vi "LoadItemValuesFromFile_Simple.vi"(0 "Array in":string[][](array[string]), 5 "FileArray":string[](array[string]), 11 "error in (no error)":errorcluster) -> (3 "Values":dbl[][](array[numeric]), 4 "Item":string[](array[string]), 6 "Time 60/min":dbl[](array[numeric]), 15 "error out":errorcluster)   [LabVIEW 2018]
doc: "Each row of the input string array specifies the Item, Dataset, Group, and Filepath of the data to be queried.\nUse these strings to look up the relevant data within the HDF5 records. The output values and corresponding TimeString or Timestamp arrays are suitable for plotting.\n\nItem (MaxValue, PeakLoc, etc.)\nDataset (Beac, Cal, etc.)\nGroup (84GHz_Cross, 72GHz_Cross, etc.)\nFile (filename of the HDF5 file)"
uses:
  <vilib>/addons/h5labview2/file/H5Fmode.ctl
  HDF5/lib_path_mod_20200519.vi
  <vilib>/addons/h5labview2/base/H5Equery.vi
  <vilib>/addons/h5labview2/attrib/H5Aread.llb/H5Aread.xnode
  <vilib>/addons/h5labview2/dataset/H5Dread.llb/H5Dread.xnode
  <vilib>/addons/h5labview2/file/H5F.lvlib
  <vilib>/addons/h5labview2/group/H5G.lvlib
  <vilib>/addons/h5labview2/dataset/H5D.lvlib
panel:
  out "UseFastRate":bool
  out "Time 1/min":dbl[](array[numeric])
  # "Item"
  # "Dataset"
  # "Group"
  # "Filepath"
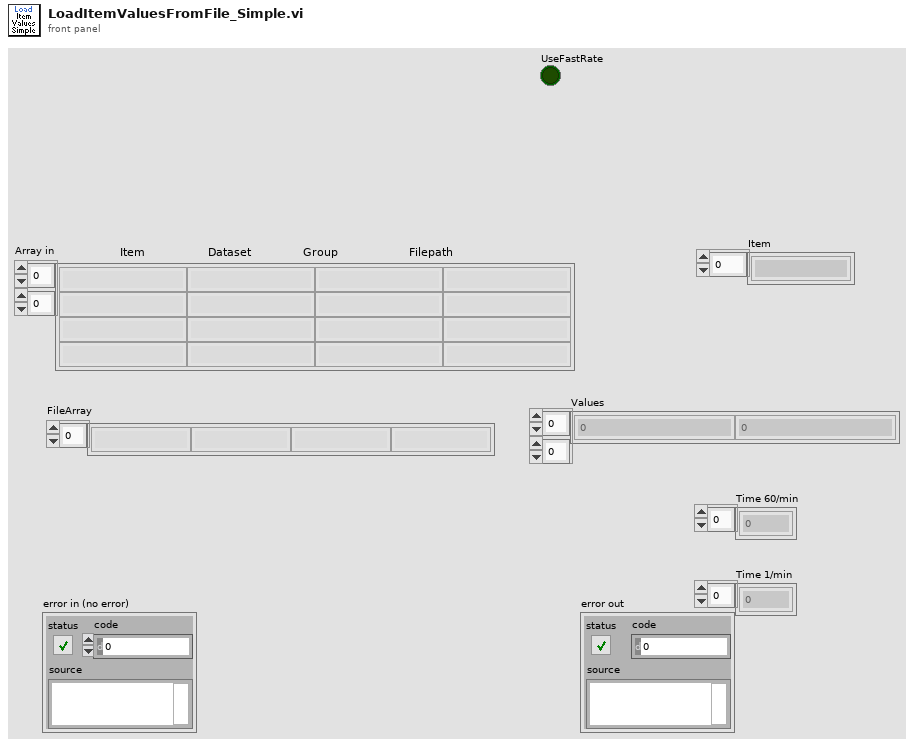
[diagram p1: front panel]
types:
  T1 = typedef "H5F.lvlib/H5Fmode.ctl" = enum16{"read-only", "read-write", "overwrite", "create new", "open or create"}
  T2 = typedef "hid_t.ctl" = i32
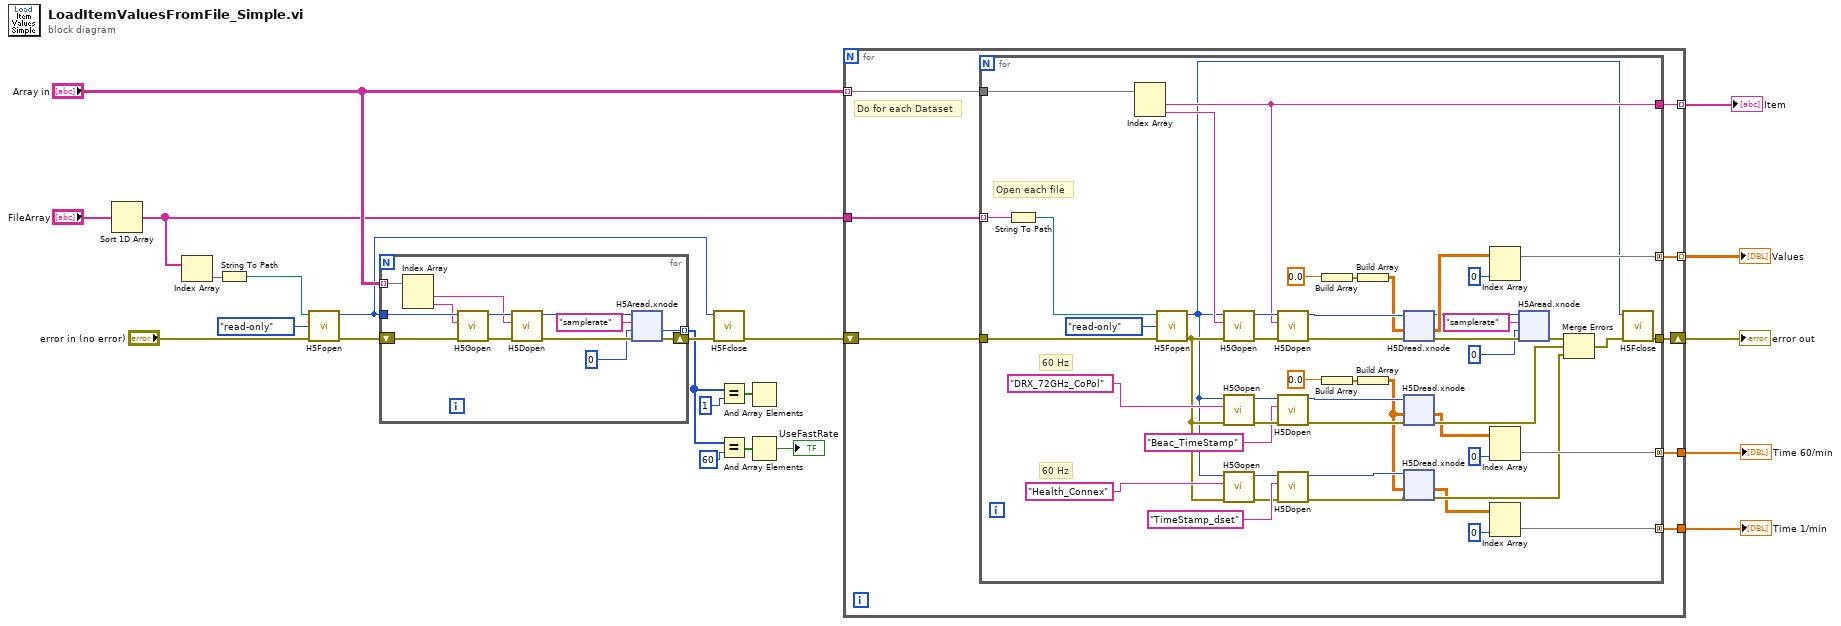
[diagram p0: block diagram]
diagram:
  n1 = Sort 1D Array(array="FileArray") -> (sorted array=w1:string[])
  n2 = Index Array(array=w1) -> (element=w15:string)  [unwired: 1 in]
  n3 = String To Path(string=w15) -> (path=w14:path)
  n4 = call <vilib>:"H5Fopen.vi"("error in (no error)"="error in (no error)", "mode (read-only)"=H5Fmode."read-only" ("mode"), "path"=w14) -> ("error out"=w11:errorcluster, "ref out"=w2:T2)  [unwired: 7 in]
  n5 = for {
    tunnel: w2 -> [w34]
    shift-right: [w28] -> w10
    shift-left: w11 -> [w31]
    tunnel: [w26] -> w7 mode=indexing
    tunnel: "Array in" -> [w25] mode=indexing
    n6 = Index Array(array=w25) -> (element #1=w23:string, element #2=w24:string)  [unwired: 2 in]
    n7 = call <vilib>:"H5Gopen.vi"("error in (no error)"=w31, "name"=w24, "ref in"=w34) -> ("error out"=w30:errorcluster, "group out"=w33:T2)  [unwired: 7 in]
    n8 = call <vilib>:"H5Dopen.vi"("error in (no error)"=w30, "name"=w23, "loc in"=w33) -> ("error out"=w29:errorcluster, "dset out"=w32:T2)  [unwired: 7 in]
    n9 = xnode "H5Aread.xnode"("error in (no error)"=w29, "default"=u32 0, "attrib name"="samplerate", "ref in"=w32) -> ("error out"=w28:errorcluster, "data"=w26:u32)  [unwired: 2 in, 2 out]
  }
  n10 = call <vilib>:"H5Fclose.vi"("error in (no error)"=w10, "ref"=w2) -> ("error out"=w13:errorcluster)  [unwired: 9 in]
  n11 = Equal?(x=w7, y=u32 1 ("data")) -> (x = y?=w5:bool[])
  n12 = Equal?(x=w7, y=u32 60 ("data")) -> (x = y?=w6:bool[])
  n13 = And Array Elements(Boolean array=w5) -> ()  [unwired: 1 out]
  n14 = And Array Elements(Boolean array=w6) -> (logical AND=→"UseFastRate":bool)
  n15 = for {
    tunnel: w1 -> [w58]
    tunnel: [w56] -> w21 mode=indexing
    shift-right: [w57] -> w22
    shift-left: w13 -> [w52]
    tunnel: [w55] -> w20
    tunnel: "Array in" -> [w54] mode=indexing
    tunnel: [w53] -> w19 mode=indexing
    tunnel: [w51] -> w18
    # "Do for each Dataset"
    n16 = for {
      tunnel: w58 -> [w106] mode=indexing
      tunnel: [w100] -> w57
      tunnel: [w94] -> w56 mode=concatenating
      tunnel: [w83] -> w55 mode=concatenating
      tunnel: w54 -> [w82]
      tunnel: [w80] -> w53
      tunnel: w52 -> [w79]
      tunnel: [w76] -> w51 mode=concatenating
      # "60 Hz"
      # "60 Hz"
      # "Open each file"
      n17 = String To Path(string=w106) -> (path=w105:path)
      n18 = Index Array(array=w82) -> (element #1=w80:string, element #2=w81:string)  [unwired: 2 in]
      n19 = call <vilib>:"H5Fopen.vi"("error in (no error)"=w79, "mode (read-only)"=H5Fmode."read-only" ("mode"), "path"=w105) -> ("error out"=w70:errorcluster, "ref out"=w68:T2)  [unwired: 7 in]
      n20 = call <vilib>:"H5Gopen.vi"("error in (no error)"=w70, "name"=w81, "ref in"=w68) -> ("error out"=w102:errorcluster, "group out"=w104:T2)  [unwired: 7 in]
      n21 = call <vilib>:"H5Gopen.vi"("error in (no error)"=w70, "name"="DRX_72GHz_CoPol", "ref in"=w68) -> ("error out"=w90:errorcluster, "group out"=w88:T2)  [unwired: 7 in]
      n22 = call <vilib>:"H5Gopen.vi"("error in (no error)"=w70, "name"="Health_Connex", "ref in"=w68) -> ("error out"=w71:errorcluster, "group out"=w72:T2)  [unwired: 7 in]
      n23 = call <vilib>:"H5Dopen.vi"("error in (no error)"=w102, "name"=w80, "loc in"=w104) -> ("error out"=w101:errorcluster, "dset out"=w103:T2)  [unwired: 7 in]
      n24 = call <vilib>:"H5Dopen.vi"("error in (no error)"=w90, "name"="Beac_TimeStamp", "loc in"=w88) -> ("error out"=w91:errorcluster, "dset out"=w89:T2)  [unwired: 7 in]
      n25 = call <vilib>:"H5Dopen.vi"("error in (no error)"=w71, "name"="TimeStamp_dset", "loc in"=w72) -> ("error out"=w69:errorcluster, "dset out"=w67:T2)  [unwired: 7 in]
      n26 = Build Array(0.0 ("HDF5_ToneInfo in")) -> (w99:dbl[])
      n27 = Build Array(0.0 ("HDF5_ToneInfo in")) -> (w92:dbl[])
      n28 = Build Array(w99) -> (w98:dbl[][])
      n29 = Build Array(w92) -> (w66:dbl[][])
      n30 = xnode "H5Dread.xnode"("error in (no error)"=w101, "default"=w98, "ref in"=w103) -> ("error out"=w62:errorcluster, "data"=w96:dbl[][], "ref out"=w63:i32)  [unwired: 3 in, 1 out]
      n31 = xnode "H5Dread.xnode"("error in (no error)"=w91, "default"=w66, "ref in"=w89) -> ("error out"=w85:errorcluster, "data"=w84:dbl[][])  [unwired: 3 in, 2 out]
      n32 = xnode "H5Dread.xnode"("error in (no error)"=w69, "default"=w66, "ref in"=w67) -> ("error out"=w65:errorcluster, "data"=w64:dbl[][])  [unwired: 3 in, 2 out]
      n33 = Index Array(array=w96, index (col)=0 ("disabled index (col)")) -> (element=w94:dbl[])  [unwired: 1 in]
      n34 = Index Array(array=w84, index (col)=0 ("disabled index (col)")) -> (element=w83:dbl[])  [unwired: 1 in]
      n35 = Index Array(array=w64, index (col)=0 ("disabled index (col)")) -> (element=w76:dbl[])  [unwired: 1 in]
      n36 = xnode "H5Aread.xnode"("error in (no error)"=w62, "default"=u32 0, "attrib name"="samplerate", "ref in"=w63) -> ("error out"=w61:errorcluster)  [unwired: 2 in, 3 out]
      n37 = Merge Errors(w61, w85, w65) -> (w86:errorcluster)
      n38 = call <vilib>:"H5Fclose.vi"("error in (no error)"=w86, "ref"=w68) -> ("error out"=w100:errorcluster)  [unwired: 9 in]
    }
  }
  "error out" <- w22
  "Item" <- w19
  "Values" <- w21
  "Time 60/min" <- w20
  "Time 1/min" <- w18
